vi "TDT-Stream DO.vi"(0 "RPcox":refnum<k7>, 2 "Action":T1=enum."Write", 5 "Restart":bool, 7 "Output array":bool[][](array[boolean]), 9 "Chans":i32[](array[numeric]), 11 "error in (no error)":errorcluster) -> (4 "RPcox thru":refnum<k7>, 15 "error out":errorcluster={"status"=FALSE, "code"=0, "source"="."})   [LabVIEW 2020]
uses:
  TDT-Signal Bank Action.ctl
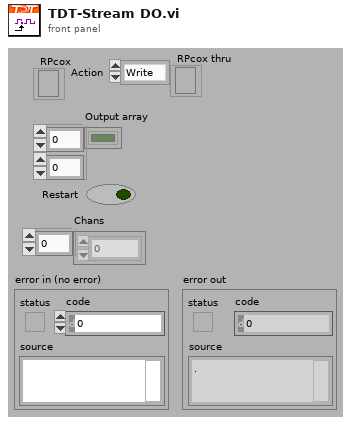
[diagram p1: front panel]
types:
  T1 = typedef "TDT-Signal Bank Action.ctl" = enum16{"Init", "Write", "Read", "Rewrite", "Reset", "Recycle", "Ramp up", "Ramp down", "Zero"}
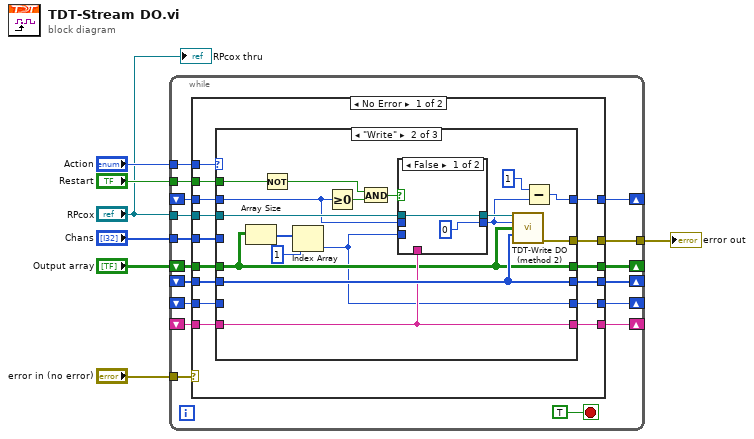
[diagram p0: block diagram]
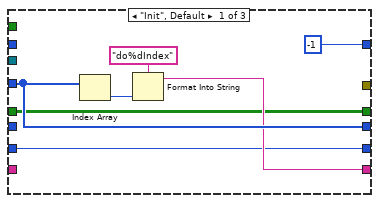
[diagram p2: hidden frame]
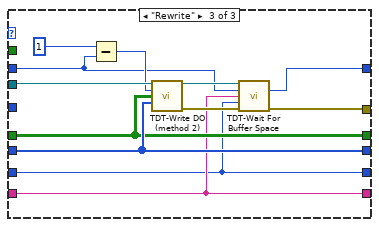
[diagram p4: hidden frame]
diagram:
  n1 = while {
    tunnel: [w24] -> w7
    tunnel: "error in (no error)" -> [w23]
    tunnel: "RPcox" -> [w22]
    tunnel: "Action" -> [w20]
    shift-right: [w18] -> _
    shift-left: _ -> [w17]
    tunnel: "Chans" -> [w16]
    shift-right: [w15] -> _
    shift-left: _ -> [w14]
    shift-right: [w13] -> _
    shift-left: _ -> [w12]
    shift-right: [w11] -> _
    shift-left: _ -> [w10]
    shift-right: [w9] -> _
    shift-left: "Output array" -> [w21]
    tunnel: "Restart" -> [w8]
    stop <- TRUE stop-if-true
    n2 = case shown="No Error" w23 {
      selector: w23 -> [_ w85]
      tunnel: [w34 w85] -> w24
      tunnel: w22 -> [w35 _]
      tunnel: w21 -> [w39 w80]
      tunnel: w20 -> [w38 _]
      tunnel: [w37 w84] -> w18
      tunnel: w17 -> [w36 w84]
      tunnel: w16 -> [w33 _]
      tunnel: [w32 w83] -> w15
      tunnel: w14 -> [w31 w83]
      tunnel: [w30 w82] -> w13
      tunnel: w12 -> [w29 w82]
      tunnel: [w28 w81] -> w11
      tunnel: w10 -> [w27 w81]
      tunnel: [w26 w80] -> w9
      tunnel: w8 -> [w25 _]
      frame No Error {
        n3 = case shown="\"Write\"" w38 {
          tunnel: w39 -> [w40 w53 w73]
          tunnel: [-1 w63 w78] -> w37
          tunnel: w36 -> [_ w57 w71]
          tunnel: w35 -> [_ w61 w76]
          tunnel: [_ w59 w68] -> w34
          tunnel: w33 -> [w44 _ _]
          tunnel: [w44 w55 w74] -> w32
          tunnel: w31 -> [_ w55 w74]
          tunnel: [w42 w54 w70] -> w30
          tunnel: w29 -> [_ w54 w70]
          tunnel: [w41 w51 w69] -> w28
          tunnel: w27 -> [w41 _ w69]
          tunnel: [w40 w53 w73] -> w26
          tunnel: w25 -> [_ w48 _]
          frame "Init", Default {
            n4 = Index Array(array=w44) -> (element=w43:i32)  [unwired: 1 in]
            n5 = Format Into String(format string="do%dIndex", w43) -> (resulting string=w42:string)  [unwired: 2 in, 1 out]
          }
          frame "Write" {
            n6 = Array Size(array=w53) -> (size(s)=w52:i32[])
            n7 = Not(x=w48) -> (.not. x?=w47:bool)
            n8 = Index Array(array=w52, index=1) -> (element=w51:i32)
            n9 = Greater Or Equal To 0?(x=w57) -> (x >= 0?=w56:bool)
            n10 = And(x=w47, y=w56) -> (x .and. y?=w49:bool)
            n11 = case shown="False" w49 {
              tunnel: w61 -> [w65 w66]
              tunnel: [w65 w66] -> w60
              tunnel: w57 -> [_ w67]
              tunnel: w51 -> [_ _]
              tunnel: [0 ("Next Buffer Out") w67] -> w58
              tunnel: w54 -> [_ _]
              frame False {
              }
              frame True {
              }
            }
            n12 = call "TDT-Write DO (method 2).vi"("RPcox"=w60, "Next Buffer"=w58, "Input array"=w53, "Chans"=w55) -> ("error out"=w59:errorcluster)  [unwired: 10 in, 1 out]
            n13 = Subtract(x=1, y=w58) -> (x-y=w63:i32)
          }
          frame "Rewrite" {
            n14 = Subtract(x=1, y=w71) -> (x-y=w75:i32)
            n15 = call "TDT-Write DO (method 2).vi"("RPcox"=w76, "Next Buffer"=w75, "Input array"=w73, "Chans"=w74) -> ("RPcox (thru)"=w72:refnum<k7>, "error out"=w77:errorcluster)  [unwired: 10 in]
            n16 = call "TDT-Wait For Buffer Space.vi"("RPcox"=w72, "Next Buffer"=w71, "Tag"=w70, "Buffer Length"=w69, "error in (no error)"=w77) -> ("Next Buffer thru"=w78:i32, "error out"=w68:errorcluster)  [unwired: 8 in, 1 out]
          }
        }
      }
      frame Error {
      }
    }
  }
  "error out" <- w7
  "RPcox thru" <- "RPcox"
